vi "期末9-test.vi"() -> ()   [LabVIEW 2014]
panel:
  out "Numeric":dbl
  in  "stop":bool
  out "Array":dbl[][](array[numeric])
  in  "Boolean":bool
  out "填入飽和磁場分量尖點座標和":dbl
  out "填入飽和磁場分量尖點座標和平均":dbl
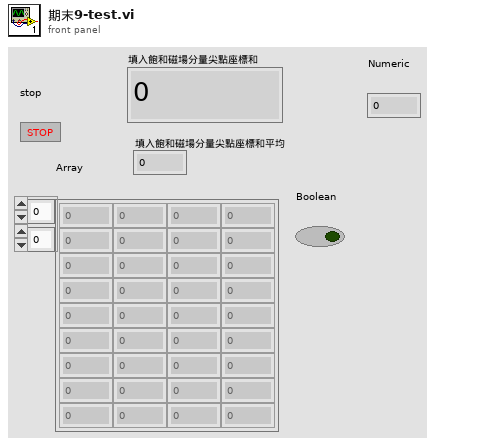
[diagram p1: front panel]
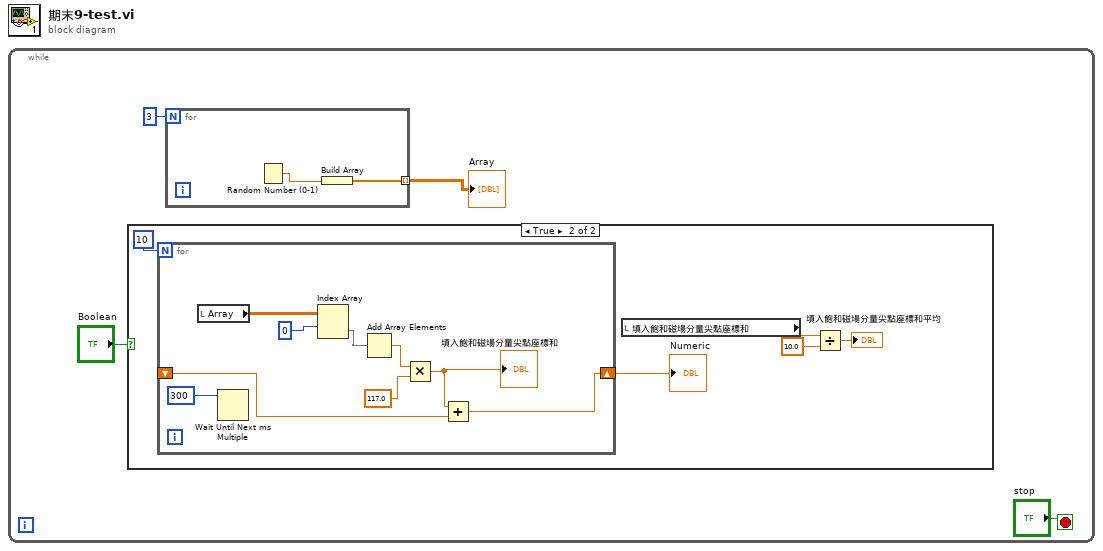
[diagram p0: block diagram]
diagram:
  n1 = while {
    stop <- "stop" stop-if-true
    n2 = case shown="True" "Boolean" {
      frame False {
      }
      frame True {
        n3 = for {
          N: 10 -> [_]
          shift-right: [w13] -> w7
          shift-left: _ -> [w15]
          n4 = local read "Array"() -> (w12:dbl[][])
          n5 = Wait Until Next ms Multiple(millisecond multiple=u32 300 ("millisecond timer value")) -> ()  [unwired: 1 out]
          n6 = Index Array(array=w12, index (row)=0) -> (element=w19:dbl[])  [unwired: 1 in]
          n7 = Add Array Elements(numeric array=w19) -> (sum=w18:dbl)
          n8 = Multiply(x=w18, y=117.0) -> (x*y=w14:dbl)
          "填入飽和磁場分量尖點座標和" <- w14
          n9 = Add(x=w14, y=w15) -> (x+y=w13:dbl)
        }
        "Numeric" <- w7
        n10 = local read "填入飽和磁場分量尖點座標和"() -> (w10:dbl)
        n11 = Divide(x=w10, y=10.0) -> (x/y=→"填入飽和磁場分量尖點座標和平均":dbl)
      }
    }
    n12 = for {
      N: 3 -> [_]
      tunnel: [w6] -> w2 mode=indexing
      n13 = Random Number (0-1)() -> (number: 0 to 1=w5:dbl)
      n14 = Build Array(w5) -> (w6:dbl[])
    }
    "Array" <- w2
  }
